vi "Launched SeqEdit.vi"(8 "error in":errorcluster, 10 "Reply Payload":T1) -> (0 "error out":errorcluster)   [LabVIEW 2025, in "TS Environment Manager.lvlib"]
doc: "This broadcast is sent after the sequence editor is launched.\n\n_____\nCreated using DQMH Framework: Event Scripter 7.1.1.1528."
uses:
  TS Environment Manager.lvlib
  Launch Sequence Editor (Reply Payload)--cluster.ctl
  Type Definitions/Architecture--enum.ctl
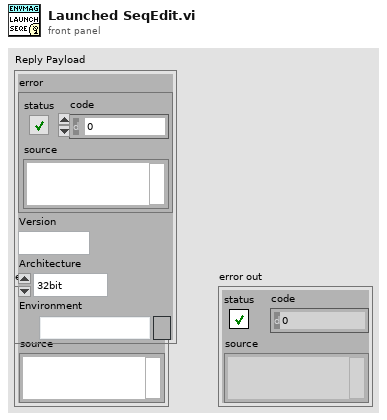
[diagram p1: front panel]
types:
  T1 = typedef "TS Environment Manager.lvlib/Launch Sequence Editor (Reply Payload)--cluster.ctl" = cluster{"error":errorcluster, "Version":string, "Architecture":T2, "Environment":path}
  T2 = typedef "Architecture--enum.ctl" = enum16{"32bit", "64bit"}
  T3 = typedef "TS Environment Manager.lvlib/Broadcast Events--cluster.ctl" = cluster{"Module Did Init":refnum<user-event>, "Status Updated":refnum<user-event>, "Error Reported":refnum<user-event>, "Module Did Stop":refnum<user-event>, "Update Module Execution Status":refnum<user-event>, "Version Activated":refnum<user-event>, "Launched SeqEdit":refnum<user-event>}
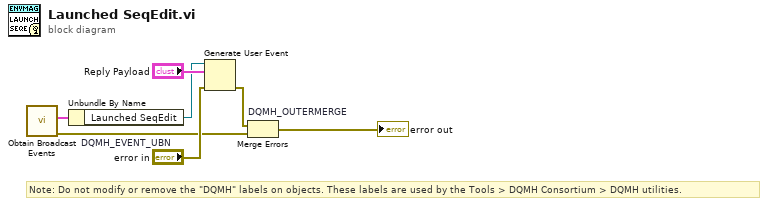
[diagram p0: block diagram]
diagram:
  # "Note: Do not modify or remove the \"DQMH\" labels on objects. These labels are used by the Tools > DQMH Consortium > DQMH utilities."
  n1 = call "Obtain Broadcast Events.vi"() -> ("error out"=w2:errorcluster, "TS Environment Manager Broadcast Events"=w1:T3)  [unwired: 10 in]
  n2 = Unbundle By Name "DQMH_EVENT_UBN"(w1) -> ("Launched SeqEdit"=w4:refnum<user-event>)
  n3 = Generate User Event(user event=w4, event data cluster="Reply Payload", error in="error in") -> (error out=w3:errorcluster)  [unwired: 1 in, 1 out]
  n4 = Merge Errors "DQMH_OUTERMERGE"(w3, w2) -> (→"error out":errorcluster)
